vi "Położenie robota z uwzględnieniem jego ewentualnej zmiany.vi"(6 "Parametry robota":T1={"Promień koła [m]"=0.045, "Szerokość robota [m]"=0.37}, 7 "Początkowa odległość robota od startu":cluster{" X [m]":dbl, "Y [m]":dbl}, 9 "Azymut robota":dbl, 10 "Prędkość kątowa prawych kół [rad/s]":dbl, 11 "Prędkość kątowa lewych kół [rad/s]":dbl) -> (0 "Zmiana położenia robota?":bool, 1 "Azymut [stopnie]":dbl, 2 "Odległość robota od startu":cluster{"X[m]":dbl, "Y[m]":dbl})   [LabVIEW 2012, in "Biblioteka moduł map v3.lvlib" / "Matematyczne.lvlib"]
uses:
  Matematyczne/Matematyczne.lvlib
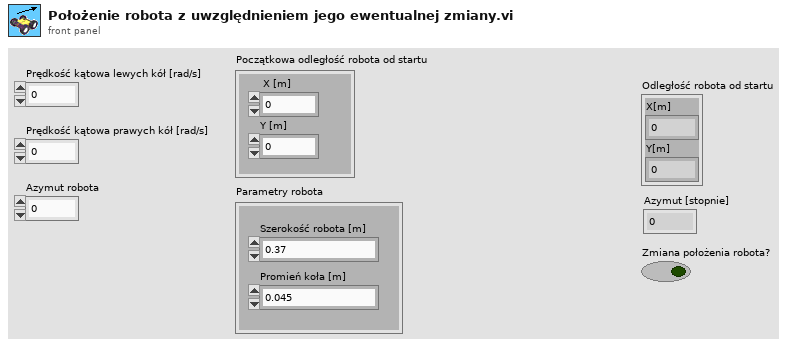
[diagram p1: front panel]
types:
  T1 = cluster{"Promień koła [m]":dbl, "Szerokość robota [m]":dbl}
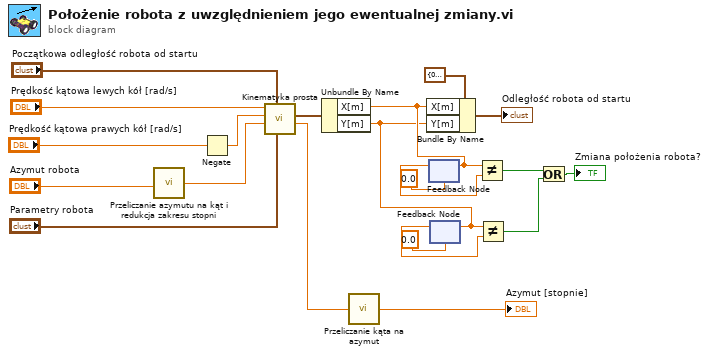
[diagram p0: block diagram]
diagram:
  n1 = call "Przeliczanie azymutu na kąt i redukcja zakresu stopni.vi"("Azymut [stoponie]"="Azymut robota") -> ("Kąt [stopnie]"=w15:dbl)  [unwired: 4 in]
  n2 = Negate(x="Prędkość kątowa prawych kół [rad/s]") -> (-x=w16:dbl)
  n3 = call "Kinematyka prosta.vi"("Parametry robota"="Parametry robota", "Początkowa odległość robota od startu"="Początkowa odległość robota od startu", "Orientacja [stopnie]"=w15, "Prędkość kątowa prawych kół [rad/s]"=w16, "Prędkość kątowa lewych kół [rad/s]"="Prędkość kątowa lewych kół [rad/s]") -> ("Orientacja kąt [stopnie]"=w12:dbl, "Odległość robota od startu"=w11:cluster{"X[m]":dbl, "Y[m]":dbl})  [unwired: 4 in]
  n4 = Unbundle By Name(w11) -> ("X[m]"=w4:dbl, "Y[m]"=w3:dbl)
  n5 = call "Przeliczanie kąta na azymut.vi"("Kąt [stoponie]"=w12) -> ("Azymut [stopnie]"=→"Azymut [stopnie]":dbl)  [unwired: 4 in]
  n6 = Bundle By Name(cluster=cluster{"X[m]":dbl, "Y[m]":dbl} {"X[m]"=0.0, "Y[m]"=0.0} ("Odległość robota od startu"), "X[m]"=w4, "Y[m]"=w3) -> (→"Odległość robota od startu":cluster{"X[m]":dbl, "Y[m]":dbl})
  n7 = feedback #1(0.0 ("Y")) -> (w7:dbl)
  n8 = feedback-in #1(w4) -> ()
  n9 = feedback #2(0.0 ("Y")) -> (w5:dbl)
  n10 = feedback-in #2(w3) -> ()
  n11 = Not Equal?(x=w4, y=w7) -> (x != y?=w2:bool)
  n12 = Not Equal?(x=w3, y=w5) -> (x != y?=w1:bool)
  n13 = Or(x=w2, y=w1) -> (x .or. y?=→"Zmiana położenia robota?":bool)
